vi "Stop Core.vi"(10 "final error code":i32, 11 "Python Protocol in":refnum<class "Python Protocol.lvclass">) -> (3 "Python Protocol out":refnum<class "Python Protocol.lvclass">)   [LabVIEW 2012, in "Python Protocol Actor.lvlib" / "Python Protocol.lvclass"]
uses:
  Python Protocol.lvclass
  <vilib>/ActorFramework/Actor/Actor.lvclass
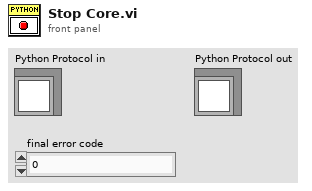
[diagram p1: front panel]
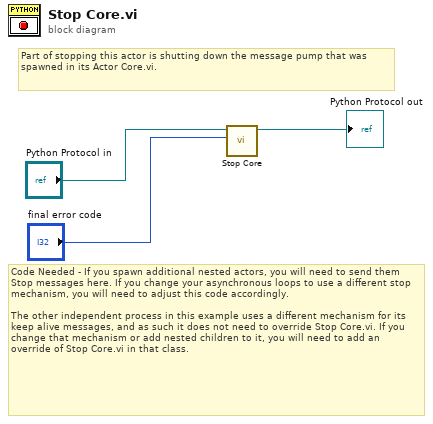
[diagram p0: block diagram]
diagram:
  # "Code Needed - If you spawn additional nested actors, you will need to send them Stop messages here. If you change your asynchronous loops to use a different stop mechanism, you will need to adjust this code accordingly.\n\nThe other independent process in this example uses a different mechanism for its keep alive messages, and as such it does not need to override Stop Core.vi. If you change that mechanism or add nested children to it, you will need to add an override of Stop Core.vi in that class."
  # "Part of stopping this actor is shutting down the message pump that was spawned in its Actor Core.vi."
  n1 = call-parent "Stop Core.vi"("final error code"="final error code", "Actor in"="Python Protocol in") -> ("Actor out"=→"Python Protocol out":refnum<class "Python Protocol.lvclass">)  [unwired: 9 in]
